vi "Global_1.vi"() -> ()   [LabVIEW 2019]
panel:
  out "Sampling Rate":dbl
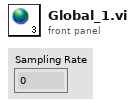
[diagram p1: front panel]
diagram:
